vi "IR-Read.vi"(7 "Reset":bool, 8 "Error In":errorcluster) -> (0 "Error Out":errorcluster, 3 "輸出紅外線值":dbl[](array[numeric]))   [LabVIEW 2019]
uses:
  <vilib>/Utility/error.llb/Error Cluster From Error Code.vi
  <vilib>/myRIO/Common/Instrument Driver Framework/myRIO v1.0/AI/vis/myRIO v1.0 Read AI.vi
  <vilib>/myRIO/Instrument Drivers/Onboard IO/AI/AI.lvlib
  <vilib>/ptbypt/NI_PtbyPt.lvlib
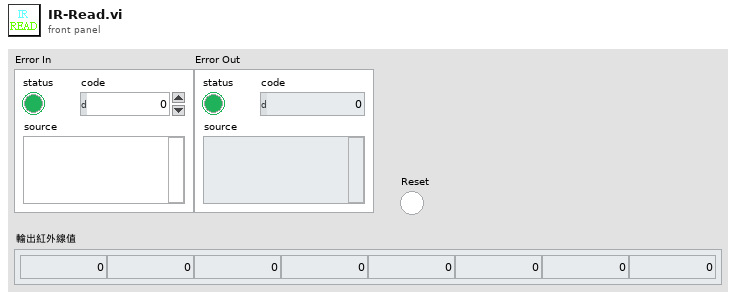
[diagram p1: front panel]
types:
  T1 = typedef "AI.lvlib/AI Reference.ctl" = cluster{"myRIO Reference":T2, "AI Channels List":T6, "AI Scaling Constants List":T8}
  T2 = typedef "myRIO Generic Hardware Reference.ctl" = cluster{"myRIO Model":T3, "myRIO Hardware Reference":T4}
  T3 = typedef "Hardware Version Enum.ctl" = enum16{"Unknown", "myRIO-1900", "myRIO-1950", "roboRIO", "NI ELVIS RIO CM", "ELVIS III"}
  T4 = typedef "myRIO v1.0 Reference.ctl" = cluster{"Generic FPGA Reference":T5, "Allow multiple opens":bool}
  T5 = typedef "Generic FPGA Reference.ctl" = refnum<k20>
  T6 = typedef "AI Channels List.ctl" = T7[]
  T7 = typedef "AI Channels Enum.ctl" = enum16{"Not Connected", "AudioIn/Left", "AudioIn/Right", "C/AI0", "C/AI1", "A/AI0", "A/AI1", "A/AI2", "A/AI3", "A/AI4", "A/AI5", "A/AI6", "A/AI7", "B/AI0", "B/AI1", "B/AI2", "B/AI3", "B/AI4", "B/AI5", "B/AI6", "B/AI7", "AI/AI0", "AI/AI1", "AI/AI2", "AI/AI3", "A/AI0 (DIFF)", "A/AI1 (DIFF)", "A/AI2 (DIFF)", "A/AI3 (DIFF)", "B/AI0 (DIFF)", "B/AI1 (DIFF)", "B/AI2 (DIFF)", "B/AI3 (DIFF)"}
  T8 = typedef "Analog Scaling Constants List.ctl" = T9[]
  T9 = typedef "Analog Scaling Constants.ctl" = cluster{"LSB Weight (Volts)":dbl, "Offset (Volts)":dbl, "Signed?":bool}
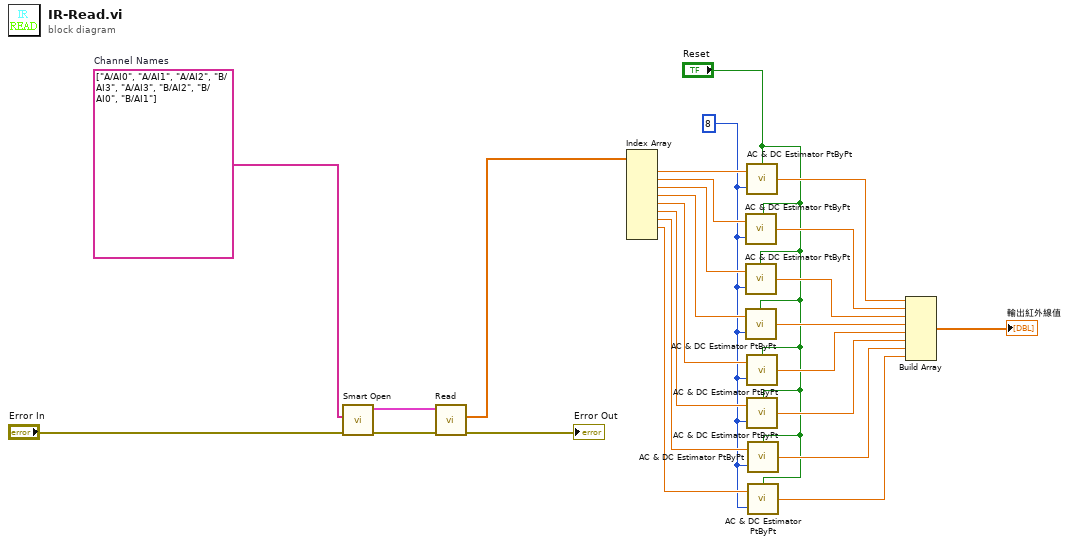
[diagram p0: block diagram]
diagram:
  w11 = 8 ("sample length")
  w25 = tag[] ["A/AI0", "A/AI1", "A/AI2", "B/AI3", "A/AI3", "B/AI2", "B/AI0", "B/AI1"]  # Channel Names
  n1 = call <vilib>:"Smart Open.vi"("error in (no error)"="Error In", "Channel Names"=w25) -> ("error out"=w22:errorcluster, "AI Ref Out"=w23:T1)  [unwired: 8 in]
  n2 = call <vilib>:"Read.vi"("error in (no error)"=w22, "AI Ref In"=w23) -> ("error out"=→"Error Out":errorcluster, "Values"=w24:dbl[])  [unwired: 7 in, 1 out]
  n3 = Index Array(array=w24) -> (element #1=w21:dbl, element #2=w20:dbl, element #3=w19:dbl, element #4=w18:dbl, element #5=w17:dbl, element #6=w16:dbl, element #7=w15:dbl, element #8=w14:dbl)  [unwired: 9 in, 1 out]
  n4 = call <vilib>:"AC & DC Estimator PtByPt.vi"("signal"=w20, "sample length"=w11, "initialize"="Reset") -> ("DC estimate (V)"=w9:dbl)  [unwired: 2 out]
  n5 = call <vilib>:"AC & DC Estimator PtByPt.vi"("signal"=w19, "sample length"=w11, "initialize"="Reset") -> ("DC estimate (V)"=w8:dbl)  [unwired: 2 out]
  n6 = call <vilib>:"AC & DC Estimator PtByPt.vi"("signal"=w18, "sample length"=w11, "initialize"="Reset") -> ("DC estimate (V)"=w7:dbl)  [unwired: 2 out]
  n7 = call <vilib>:"AC & DC Estimator PtByPt.vi"("signal"=w21, "sample length"=w11, "initialize"="Reset") -> ("DC estimate (V)"=w10:dbl)  [unwired: 2 out]
  n8 = call <vilib>:"AC & DC Estimator PtByPt.vi"("signal"=w17, "sample length"=w11, "initialize"="Reset") -> ("DC estimate (V)"=w6:dbl)  [unwired: 2 out]
  n9 = call <vilib>:"AC & DC Estimator PtByPt.vi"("signal"=w16, "sample length"=w11, "initialize"="Reset") -> ("DC estimate (V)"=w5:dbl)  [unwired: 2 out]
  n10 = call <vilib>:"AC & DC Estimator PtByPt.vi"("signal"=w15, "sample length"=w11, "initialize"="Reset") -> ("DC estimate (V)"=w4:dbl)  [unwired: 2 out]
  n11 = call <vilib>:"AC & DC Estimator PtByPt.vi"("signal"=w14, "sample length"=w11, "initialize"="Reset") -> ("DC estimate (V)"=w3:dbl)  [unwired: 2 out]
  n12 = Build Array(w10, w9, w8, w7, w6, w5, w4, w3) -> (→"輸出紅外線值":dbl[])
